vi "SetupAutonConfigFiles.vi"   [LabVIEW 2014]
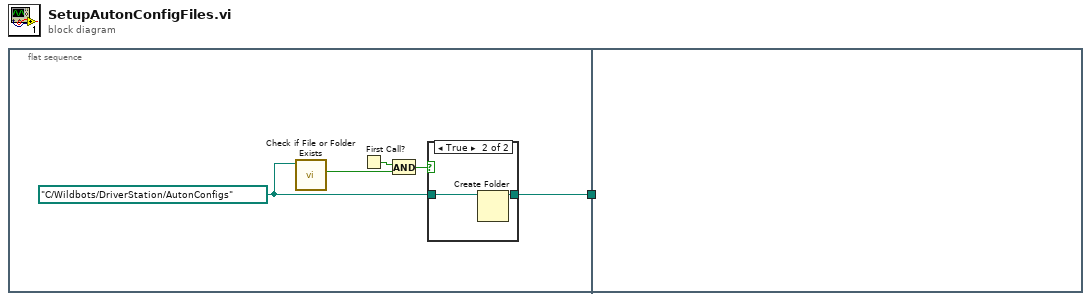
[diagram p0: block diagram]
diagram:
  n1 = flat-sequence {
    tunnel: [w2] -> w1
    tunnel: w1 -> [_]
    frame #0 {
      w3 = path "C:/Wildbots/DriverStation/AutonConfigs" ("path")
      n2 = call <vilib>:"Check if File or Folder Exists.vi"("path"=w3) -> ("file or folder exists?"=w5:bool)  [unwired: 8 in, 2 out]
      n3 = First Call?() -> (First Call?: T/F=w6:bool)
      n4 = And(x=w6, y=w5) -> (x .and. y?=w4:bool)
      n5 = case shown="True" w4 {
        tunnel: w3 -> [w7 w9]
        tunnel: [w7 w8] -> w2
        frame False {
        }
        frame True {
          n6 = Create Folder(path (use dialog)=w9) -> (created path=w8:path)  [unwired: 2 in, 2 out]
        }
      }
    }
    frame #1 {
    }
  }
